vi "DAQmx Create Channel (AI-Velocity-IEPE Sensor).vi"(0 "task in":refnum<k21>, 1 "maximum value":dbl=50.0 format="%0.2f", 2 "minimum value":dbl=-50.0 format="%0.2f", 3 "input terminal configuration":i32(ring)=-1 items=["default"=-1, "RSE"=10083, "NRSE"=10078, "Differential"=10106, "Pseudodifferential"=12529], 5 "physical channels":tag, 6 "current excitation source":i32(ring)=10200 items=["Internal"=10200, "External"=10167, "None"=10230], 7 "name to assign":string, 8 "current excitation value":dbl=0.002, 9 "units":i32(ring)=15960 items=["in/s"=15960, "m/s"=15959, "From Custom Scale"=10065], 11 "error in":errorcluster, 12 "custom scale name":tag, 13 "sensitivity":dbl=100.0, 14 "sensitivity units":i32(ring)=15964 items=["mVolts/in/s"=15964, "mVolts/mm/s"=15963]) -> (4 "task out":refnum<k21>, 15 "error out":errorcluster)   [LabVIEW 2018]
doc: "Creates channel(s) that use an IEPE velocity sensor to measure velocity."
uses:
  nilvaiu.dll
panel:
  # "input limits"
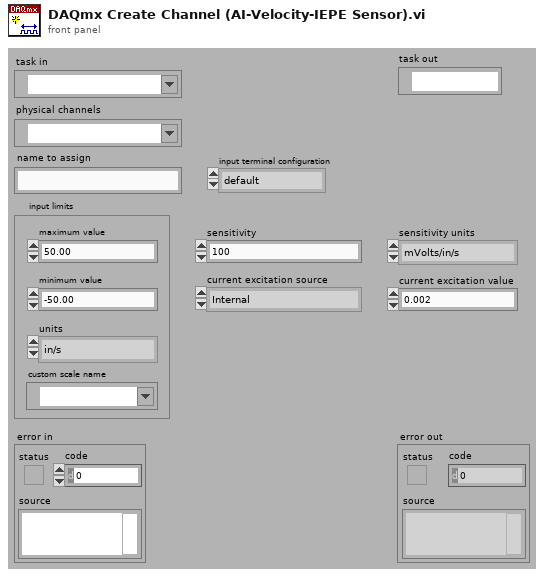
[diagram p1: front panel]
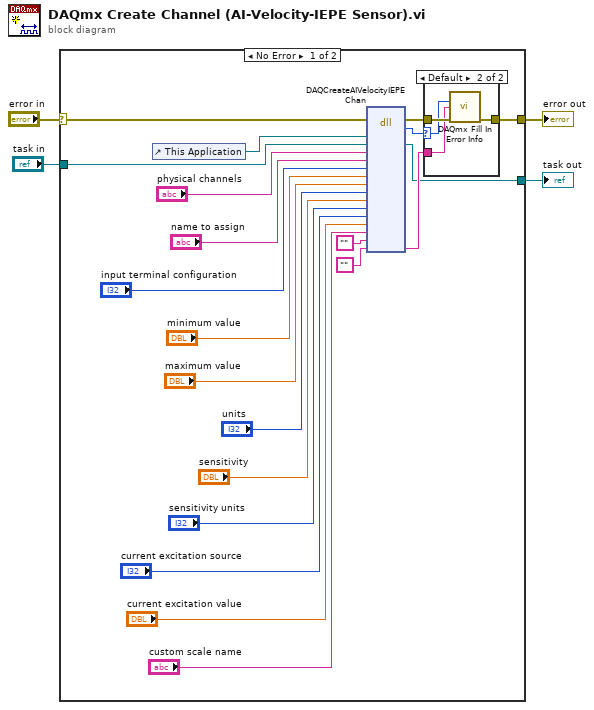
[diagram p0: block diagram]
diagram:
  n1 = case shown="No Error" "error in" {
    selector: "error in" -> [w8 w31]
    tunnel: "task in" -> [w10 w32]
    tunnel: [w9 w32] -> w3
    tunnel: [w7 w31] -> w1
    frame No Error {
      n2 = control-ref of="This Application"() -> (w11:refnum<vi>)
      n3 = dll-call lib="nilvaiu.*" fn="DAQCreateAIVelocityIEPEChan"(error in=w8, "lvAppRef"=w11, "refObjPtr"=w10, "physicalChannelName"="physical channels", "channelNameIn"="name to assign", "terminalConfig"="input terminal configuration", "minVal"="minimum value", "maxVal"="maximum value", "units"="units", "sensitivity"="sensitivity", "sensitivityUnits"="sensitivity units", "excitSource"="current excitation source", "excitVal"="current excitation value", "customScaleName"="custom scale name", "channelnamesOut"="", "extendedErrorInfo"="") -> (error out=w25:errorcluster, "return type"=w24:i32, "refObjPtr"=w9:refnum<k21>, "extendedErrorInfo"=w23:string)  [unwired: 15 in, 1 out]
      n4 = case shown="Default" w24 {
        selector: w24 -> [_ w28]
        tunnel: w25 -> [w26 w30]
        tunnel: [w26 w29] -> w7
        tunnel: w23 -> [_ w27]
        frame 0 {
        }
        frame Default {
          n5 = call "DAQmx Fill In Error Info.vi"("status code"=w28, "extended error info"=w27, "error in"=w30) -> ("error out"=w29:errorcluster)  [unwired: 1 in, 11 out]
        }
      }
    }
    frame Error {
    }
  }
  "task out" <- w3
  "error out" <- w1
